vi "Limelight_2020.vi"() -> ()   [LabVIEW 2019]
uses:
  <vilib>/Rock Robotics/Network Tables/NT Read Number.vi
  <vilib>/Rock Robotics/WPI/ThirdParty/Phoenix-LabVIEW/Motor Controller/Get/CTRE_Phoenix_MotorController_GetQuadratureData.vi
  <vilib>/Rock Robotics/Network Tables/NT Write Number.vi
panel:
  out "RPM":dbl
  out "Distance Inches":dbl
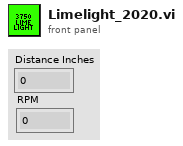
[diagram p1: front panel]
types:
  T1 = typedef "WPI_MotorControlDeviceRef.ctl" = cluster{"DeviceStatus":errorcluster, "Type":T2, "PWM":cluster{"PWM Channel":T3, "DeadBand":T4}, "CAN":cluster{"Device Number":u8, "SetOutput VI Ref":variant, "GetOutput VI Ref":variant, "Enable VI Ref":variant, "Disable VI Ref":variant, "Data":variant}, "Invert":bool, "DIO PWM":cluster{"PWM \"Enable\" Channel":T3, "DIOChannel":T5, "PWM Rate":dbl}}
  T2 = typedef "WPI_MotorControlType.ctl" = enum16{"PWM", "CAN", "DIO PWM"}
  T3 = typedef "FPGA_DIOPWMChannel.ctl" = enum8{"PWM 0", "PWM 1", "PWM 2", "PWM 3", "PWM 4", "PWM 5", "PWM 6", "PWM 7", "PWM 8", "PWM 9", "PWM MXP 0", "PWM MXP 1", "PWM MXP 2", "PWM MXP 3", "PWM MXP 4", "PWM MXP 5", "PWM MXP 6", "PWM MXP 7", "PWM MXP 8", "PWM MXP 9", "Invalid"}
  T4 = typedef "WPI_PWMDeadband.ctl" = cluster{"Name":string, "maxPositivePwm":i32, "minPositivePwm":i32, "centerPwm":i32, "maxNegativePwm":i32, "minNegativePwm":i32, "angularRange":u16}
  T5 = typedef "FPGA_DIOChannel.ctl" = enum8{"DIO 0", "DIO 1", "DIO 2", "DIO 3", "DIO 4", "DIO 5", "DIO 6", "DIO 7", "DIO 8", "DIO 9", "DIO MXP 0", "DIO MXP 1", "DIO MXP 2", "DIO MXP 3", "DIO MXP 4", "DIO MXP 5", "DIO MXP 6", "DIO MXP 7", "DIO MXP 8", "DIO MXP 9", "DIO MXP 10", "DIO MXP 11", "DIO MXP 12", "DIO MXP 13", "DIO MXP 14", "DIO MXP 15", "SPI Port CS1", "SPI Port CS2", "SPI Port CS3", "SPI Port MISO", "SPI Port MOSI", "Invalid"}
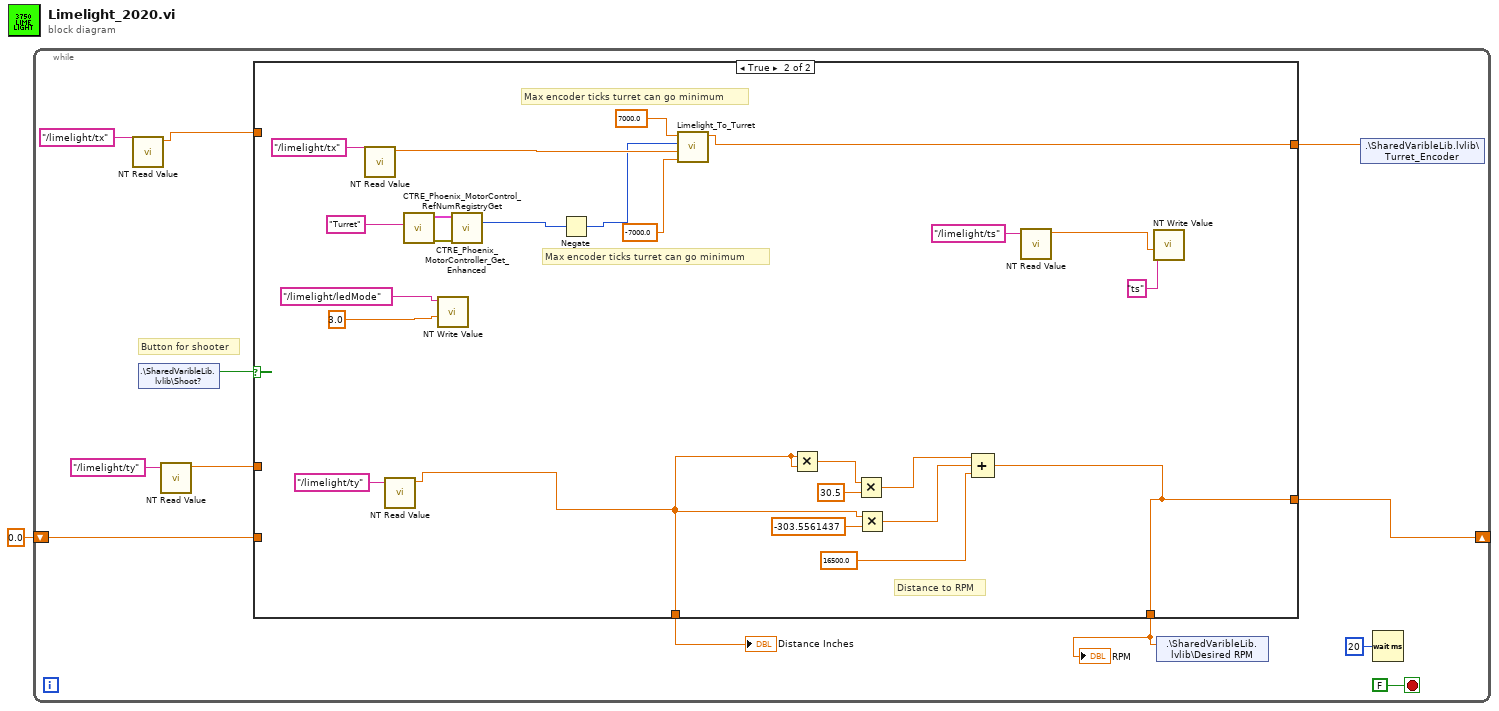
[diagram p0: block diagram]
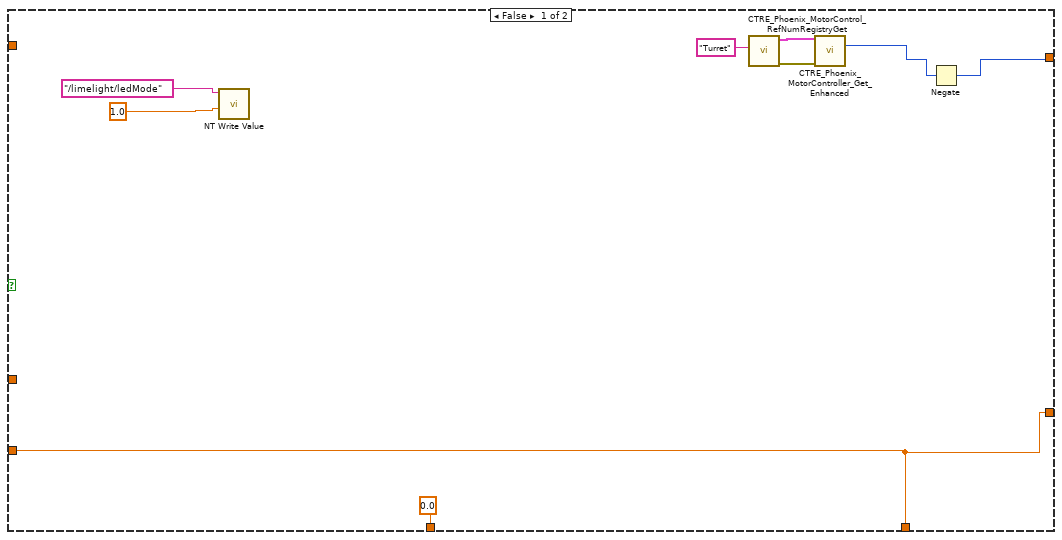
[diagram p2: hidden frame]
diagram:
  n1 = while {
    shift-right: [w4] -> _
    shift-left: 0.0 -> [w3]
    stop <- FALSE stop-if-true
    # "Button for shooter"
    n2 = call-poly <vilib>:"NT Read Value.vi"("Name"="/limelight/tx") -> ("Numeric"=w8:dbl)  [unwired: 9 in, 1 out]
    n3 = shared-variable ".\\SharedVaribleLib.lvlib\\Shoot?"() -> (w10:bool)  [unwired: 1 in, 1 out]
    n4 = call-poly <vilib>:"NT Read Value.vi"("Name"="/limelight/ty") -> ("Numeric"=w6:dbl)  [unwired: 9 in, 1 out]
    n5 = case shown="True" w10 {
      tunnel: [0.0 ("y") w29] -> w11
      tunnel: [w16 w36] -> w2
      tunnel: w8 -> [_ _]
      tunnel: w6 -> [_ _]
      tunnel: [w18 w23] -> w5
      tunnel: [w18 w23] -> w4
      tunnel: w3 -> [w18 _]
      frame False {
        n6 = call-poly <vilib>:"NT Write Value.vi"("Numeric"=1.0 ("Default Value"), "Name"="/limelight/ledMode") -> ()  [unwired: 9 in, 1 out]
        n7 = call <vilib>:"CTRE_Phoenix_MotorControl_RefNumRegistryGet.vi"("refnum name"="Turret") -> ("error out"=w19:errorcluster, "PhoenixMotorControlDevRef"=w20:T1)  [unwired: 9 in]
        n8 = call-poly <vilib>:"CTRE_Phoenix_MotorController_Get_Enhanced.vi"("PhoenixMotorControlDevRef"=w20, "error in"=w19) -> ("Quadrature Position"=w17:i32)  [unwired: 10 in, 3 out]
        n9 = Negate(x=w17) -> (-x=w16:i32)
      }
      frame True {
        # "Max encoder ticks turret can go minimum"
        # "Max encoder ticks turret can go minimum"
        # "Distance to RPM"
        n10 = call-poly <vilib>:"NT Read Value.vi"("Name"="/limelight/tx") -> ("Numeric"=w37:dbl)  [unwired: 9 in, 1 out]
        n11 = call-poly <vilib>:"NT Read Value.vi"("Name"="/limelight/ty") -> ("Numeric"=w29:dbl)  [unwired: 9 in, 1 out]
        n12 = call <vilib>:"CTRE_Phoenix_MotorControl_RefNumRegistryGet.vi"("refnum name"="Turret") -> ("error out"=w42:errorcluster, "PhoenixMotorControlDevRef"=w43:T1)  [unwired: 9 in]
        n13 = call-poly <vilib>:"NT Write Value.vi"("Numeric"=3.0 ("Default Value"), "Name"="/limelight/ledMode") -> ()  [unwired: 9 in, 1 out]
        n14 = call-poly <vilib>:"CTRE_Phoenix_MotorController_Get_Enhanced.vi"("PhoenixMotorControlDevRef"=w43, "error in"=w42) -> ("Quadrature Position"=w25:i32)  [unwired: 10 in, 3 out]
        n15 = Negate(x=w25) -> (-x=w24:i32)
        n16 = call "Limelight_To_Turret.vi"("lower limit"=-7000.0, "Limelight X"=w37, "Current"=w24, "upper limit"=7000.0) -> ("OutputForTurret"=w36:dbl)  [unwired: 7 in]
        n17 = Multiply(x=w29, y=w29) -> (x*y=w31:dbl)
        n18 = Multiply(x=w31, y=30.5) -> (x*y=w30:dbl)
        n19 = Multiply(x=w29, y=-303.5561437) -> (x*y=w41:dbl)
        n20 = Compound Arithmetic op=ADD(w30, w41, 16500.0 ("x")) -> (w23:dbl)
        n21 = call-poly <vilib>:"NT Read Value.vi"("Name"="/limelight/ts") -> ("Numeric"=w27:dbl)  [unwired: 9 in, 1 out]
        n22 = call-poly <vilib>:"NT Write Value.vi"("Numeric"=w27, "Name"="ts") -> ()  [unwired: 9 in, 1 out]
      }
    }
    "Distance Inches" <- w11
    "RPM" <- w5
    n23 = shared-variable ".\\SharedVaribleLib.lvlib\\Desired RPM"(w5) -> ()  [unwired: 1 in, 1 out]
    n24 = shared-variable ".\\SharedVaribleLib.lvlib\\Turret_Encoder"(w2) -> ()  [unwired: 1 in, 1 out]
    n25 = Wait (ms)(milliseconds to wait=u32 20) -> ()  [unwired: 1 out]
  }
